vi "Import from ProjFile VI Entry.vi"(8 "error in (no error)":errorcluster, 9 "LangFile ref":refnum<data-value>, 10 "VI Data":T1, 11 "LVProject File Path (Absolute)":path) -> (0 "error out":errorcluster, 3 "LanguageData out":refnum<class "VI Data.lvclass">)   [LabVIEW 2013, in "SET Project Data.lvlib" / "VI Data.lvclass"]
uses:
  VI Data.lvclass
  Types/ProjFile_VI Data.ctl
  Types/ProjFile_GObject Data.ctl
  Resource Data Class/Resource Data.lvclass
  VI Data.lvclass/VI Data.ctl
  Control Classes/GObject/GObject.lvclass
  SET Project Data.lvlib
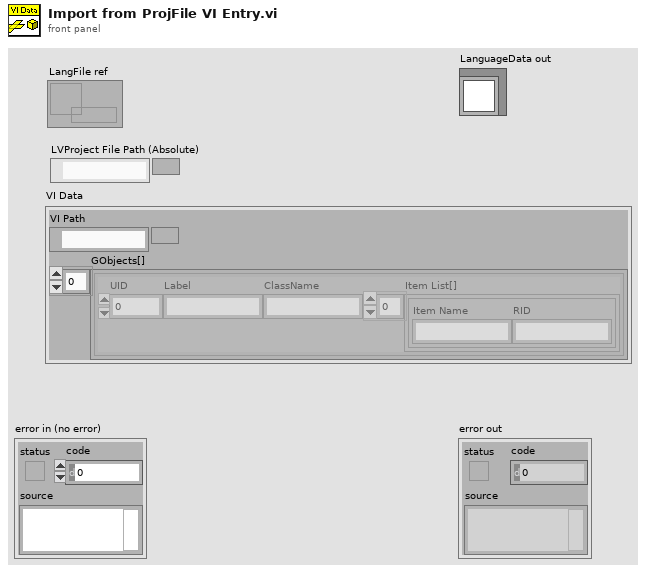
[diagram p1: front panel]
types:
  T1 = typedef "SET Project Data.lvlib/ProjFile_VI Data.ctl" = cluster{"VI Path":path, "GObjects[]":T2[]}
  T2 = typedef "SET Project Data.lvlib/ProjFile_GObject Data.ctl" = cluster{"UID":i32, "Label":string, "ClassName":string, "Item List[]":cluster{"Item Name":string, "RID":string}[]}
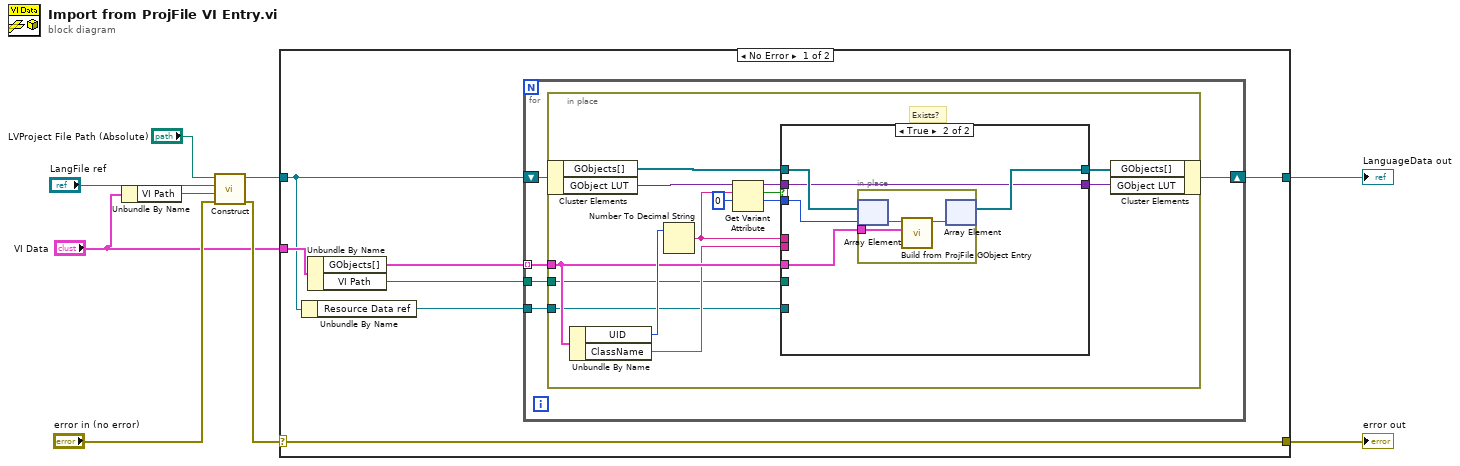
[diagram p0: block diagram]
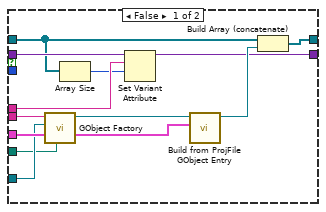
[diagram p2: hidden frame]
diagram:
  n1 = Unbundle By Name("VI Data") -> ("VI Path"=w2:path)
  n2 = call "Construct.vi"("error in (no error)"="error in (no error)", "VI Path (Relative)"=w2, "Resource Data ref"="LangFile ref", "LVProject File Path (Absolute)"="LVProject File Path (Absolute)") -> ("error out"=w6:errorcluster, "VI Data out"=w7:refnum<class "VI Data.lvclass">)  [unwired: 6 in]
  n3 = case shown="No Error" w6 {
    selector: w6 -> [w16 w57]
    tunnel: [w16 w57] -> w9
    tunnel: [w13 w56] -> w8
    tunnel: w7 -> [w10 w56]
    tunnel: "VI Data" -> [w15 _]
    frame No Error {
      n4 = Unbundle By Name(w10) -> ("Resource Data ref"=w12:refnum<data-value>)
      n5 = Unbundle By Name(w15) -> ("GObjects[]"=w14:T2[], "VI Path"=w11:path)
      n6 = for {
        shift-right: [w19] -> w13
        shift-left: w10 -> [w20]
        tunnel: w14 -> [w21] mode=indexing
        tunnel: w12 -> [w18]
        tunnel: w11 -> [w17]
        n7 = in-place {
          in-place-border: w21 -> [w26]
          in-place-border: w18 -> [w23]
          in-place-border: w17 -> [w22]
          # "Exists?"
          n8 = in-place-cluster #1(w20) -> ("GObjects[]"=w31:refnum<class "GObject.lvclass">[], "GObject LUT"=w29:variant)
          n9 = Unbundle By Name(w26) -> ("UID"=w27:i32, "ClassName"=w25:string)
          n10 = Number To Decimal String(number=w27) -> (decimal integer string=w24:string)  [unwired: 1 in]
          n11 = Get Variant Attribute(Variant=w29, name=w24, default value (empty Variant)=0) -> (duplicate Variant=w33:variant, found=w34:bool, value=w32:i32)  [unwired: 1 in, 1 out]
          n12 = case shown="True" w34 {
            tunnel: w33 -> [w47 w48]
            tunnel: w31 -> [w44 w51]
            tunnel: w32 -> [_ w49]
            tunnel: w26 -> [w42 w52]
            tunnel: w24 -> [w46 _]
            tunnel: [w41 w50] -> w30
            tunnel: [w40 w48] -> w28
            tunnel: w25 -> [w39 _]
            tunnel: w23 -> [w37 _]
            tunnel: w22 -> [w36 _]
            frame False {
              n13 = call "GObject Factory.vi"("Owning VI"=w36, "LangFile ref"=w37, "ClassName"=w39) -> ("GObject"=w38:refnum<class "GObject.lvclass">)  [unwired: 8 in]
              n14 = Array Size(array=w44) -> (size(s)=w45:i32)
              n15 = Set Variant Attribute(Variant=w47, name=w46, value=w45) -> (Variant out=w40:variant)  [unwired: 1 in, 2 out]
              n16 = call "Build from ProjFile GObject Entry.vi"("ProjFile Entry"=w42, "GObject in"=w38) -> ("GObject out"=w43:refnum<class "GObject.lvclass">)  [unwired: 8 in, 1 out]
              n17 = Build Array (concatenate)(w44, w43) -> (w41:refnum<class "GObject.lvclass">[])
            }
            frame True {
              n18 = in-place {
                in-place-border: w52 -> [w55]
                n19 = in-place-array #2(w51, w49) -> (w54:refnum<class "GObject.lvclass">)
                n20 = call "Build from ProjFile GObject Entry.vi"("ProjFile Entry"=w55, "GObject in"=w54) -> ("GObject out"=w53:refnum<class "GObject.lvclass">)  [unwired: 8 in, 1 out]
                n21 = in-place-array #2(w53) -> (w50:refnum<class "GObject.lvclass">[])  [unwired: 1 out]
              }
            }
          }
          n22 = in-place-cluster #1("GObjects[]"=w30, "GObject LUT"=w28) -> (w19:refnum<class "VI Data.lvclass">)
        }
      }
    }
    frame Error {
    }
  }
  "error out" <- w9
  "LanguageData out" <- w8
